vi "Limit Value by Threshold.vi"(1 "Threshold":dbl, 2 "Input Value":dbl) -> (0 "Output Value":dbl)   [LabVIEW 2013]
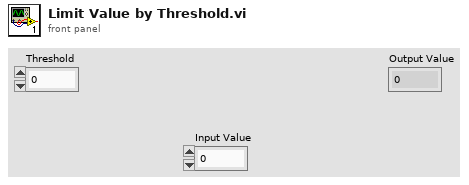
[diagram p1: front panel]
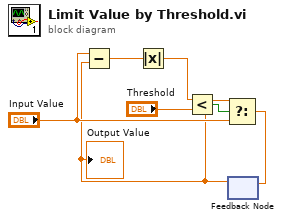
[diagram p0: block diagram]
diagram:
  n1 = feedback #1() -> (w1:dbl)  [unwired: 1 in]
  "Output Value" <- w1
  n2 = Subtract(x="Input Value", y=w1) -> (x-y=w7:dbl)
  n3 = Absolute Value(x=w7) -> (abs(x)=w6:dbl)
  n4 = Less?(x=w6, y="Threshold") -> (x < y?=w4:bool)
  n5 = Select(t=w1, s=w4, f="Input Value") -> (s? t:f=w3:dbl)
  n6 = feedback-in #1(w3) -> ()
